vi "sub_getPotentialGuesses.vi"(9 "invalid guesses":T1[](array[typedef]), 10 "current guess queue":T1[](array[typedef]), 11 "solver array":cluster{"solved":bool, "values":string[]}[][](array[cluster])) -> (1 "no valid guesses ?":bool, 2 "next guess":T1)   [LabVIEW 2018]
uses:
  guess.ctl
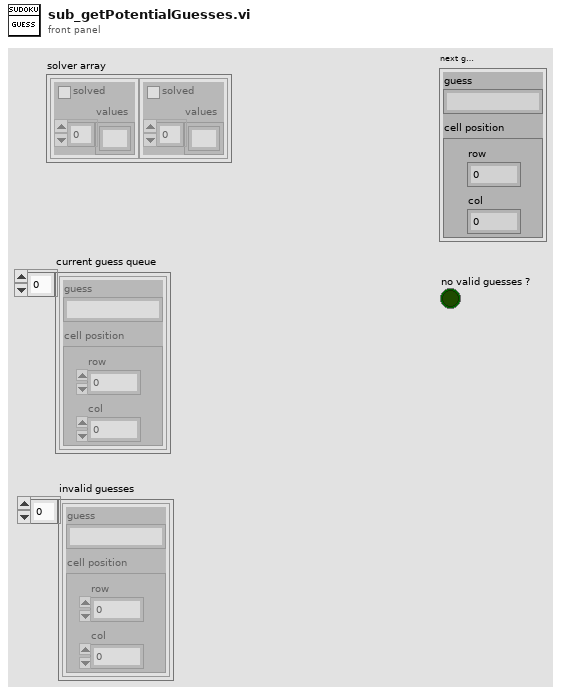
[diagram p1: front panel]
types:
  T1 = typedef "guess.ctl" = cluster{"cell position":cluster{"row":i32, "col":i32}, "guess":string}
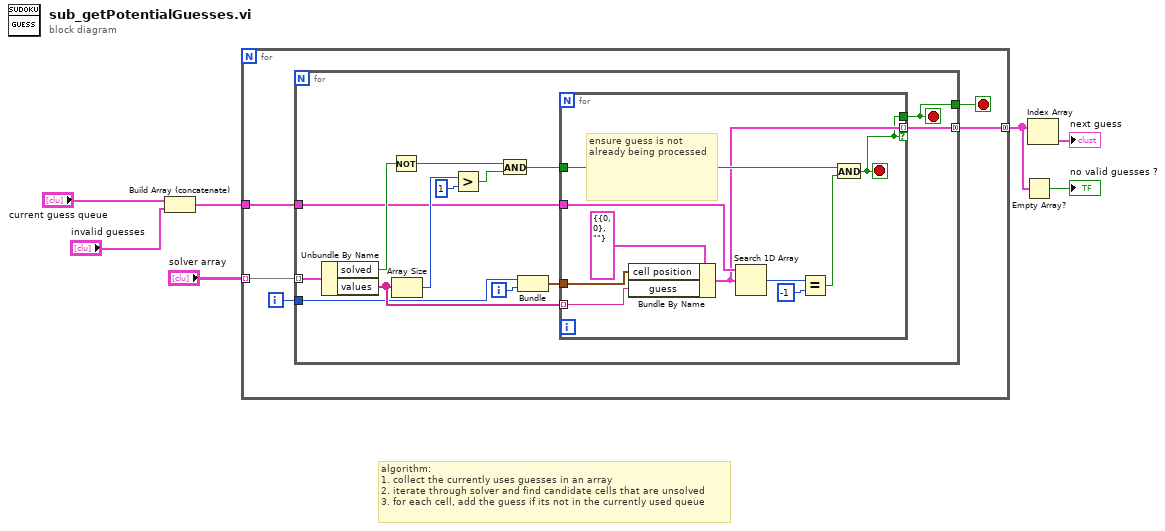
[diagram p0: block diagram]
diagram:
  # "algorithm:\n1. collect the currently uses guesses in an array\n2. iterate through solver and find candidate cells that are unsolved\n3. for each cell, add the guess if its not in the currently used queue"
  n1 = Build Array (concatenate)("current guess queue", "invalid guesses") -> (w4:T1[])
  n2 = for {
    tunnel: "solver array" -> [w12] mode=indexing
    tunnel: w4 -> [w10]
    tunnel: [w8] -> w2 mode=concatenating
    i -> [w11]
    stop <- w9 stop-if-true
    n3 = for {
      tunnel: w12 -> [w26] mode=indexing
      tunnel: w11 -> [w23]
      tunnel: w10 -> [w15]
      tunnel: [w14] -> w9
      tunnel: [w13] -> w8 mode=concatenating
      i -> [w24]
      stop <- w14 stop-if-true
      n4 = Unbundle By Name(w26) -> ("solved"=w21:bool, "values"=w25:string[])
      n5 = Not(x=w21) -> (.not. x?=w19:bool)
      n6 = Array Size(array=w25) -> (size(s)=w18:i32)
      n7 = Greater?(x=w18, y=1) -> (0:w16:bool)
      n8 = And(x=w19, y=w16) -> (x .and. y?=w20:bool)
      n9 = Bundle(w23, w24) -> (w22:cluster{i32, i32})  [unwired: 1 in]
      n10 = for {
        tunnel: w25 -> [w34] mode=indexing
        tunnel: w22 -> [w35]
        tunnel: w20 -> [w29]
        tunnel: w15 -> [w33]
        tunnel: [w28] -> w13 mode=indexing if=w27
        tunnel: [w27] -> w14
        stop <- w27 stop-if-true
        # "ensure guess is not \nalready being processed"
        n11 = Bundle By Name(cluster=T1 {"cell position"={"row"=0, "col"=0}, "guess"=""} ("guess"), "cell position"=w35, "guess"=w34) -> (w28:T1)
        n12 = Search 1D Array(1D array=w33, element=w28) -> (index of element=w32:i32)  [unwired: 1 in]
        n13 = Equal?(x=w32, y=-1) -> (x = y?=w30:bool)
        n14 = And(x=w29, y=w30) -> (x .and. y?=w27:bool)
      }
    }
  }
  n15 = Empty Array?(array=w2) -> (empty?=→"no valid guesses ?":bool)
  n16 = Index Array(array=w2) -> (element=→"next guess":T1)  [unwired: 1 in]
